vi "Handle Filling.vi"(8 "error in (no error)":errorcluster, 11 "Stand in":refnum<class "Stand.lvclass">) -> (0 "error out":errorcluster, 3 "Stand out":refnum<class "Stand.lvclass">)   [LabVIEW 2019, in "Stand.lvclass"]
uses:
  Stand.lvclass
  D:/GIT H4000/H4000/src/Device_class/Device.lvclass
  Stand.lvclass/Stand.ctl
  Device_class/Device.lvclass/Device.ctl
  FPGA/TypeDef/DO index.ctl
  TypeDef/Direction.ctl
  FPGA/TypeDef/AI index.ctl
  AI_class/AI.lvclass/AI.ctl
  AnalogComparator_class/AnalogComparator.lvclass/AnalogComparator.ctl
  TypeDef/Step_Name.ctl
  TypeDef/Active Motor.ctl
  TypeDef/Motor N.ctl
  f638fa31-f737-482a-bde8-81f5a2056bae.vi
  AnalogComparator_class/GetStatus.vi
  FPGA_API_class/FPGA API.lvclass
  Device_class/Device.lvclass
  PM_Group_class/PM_Group.lvclass
  AI_class/AI.lvclass
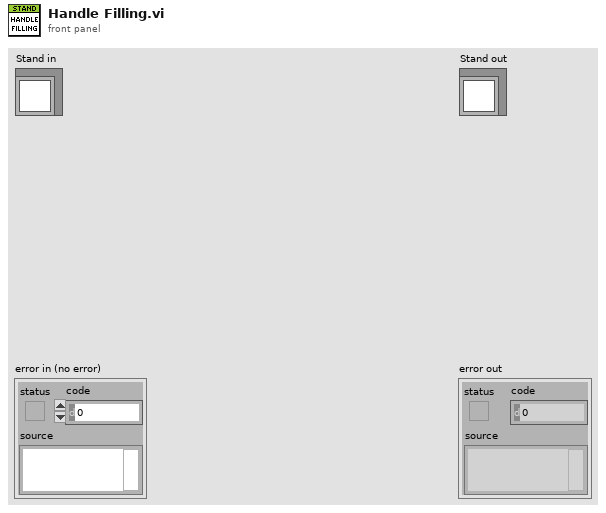
[diagram p1: front panel]
types:
  T1 = typedef "Step_Name.ctl" = enum16{"NONE", "Filling DUT", "Filling Chamber", "Pressure Up DUT", "Abrupt Pressure Release DUT", "Smooth Pressure Release DUT", "Pressure Up Chamber", "Abrupt Pressure Release Chamber", "Smooth Pressure Release Chamber", "Measuring leakage sensor 41.3", "Measuring leakage burette 42", "Low Pressure DUT", "Low Pressure Chamber", "Low Pressure HPP", "ALARM", "Open Air", "MicroStep DUT", "MicroStep CMBR"}
  T2 = typedef "Direction.ctl" = enum16{"None", "Chamber", "DUT"}
  T3 = typedef "Active Motor.ctl" = cluster{"Active":bool, "MotorN":T4}
  T4 = typedef "Motor N.ctl" = enum16{"M12", "M21", "M24"}
  T5 = typedef "AI index.ctl" = u8
  T6 = typedef "DO index.ctl" = u8
  T7 = typedef "AI_Data.ctl" = cluster{"Stat Data":T8, "OutOfRangeMax":bool, "OutOfRangeMin":bool, "HIHI":bool, "HI":bool, "LO":bool, "LOLO":bool}
  T8 = typedef "AI Statistics Data.ctl" = cluster{"raw mean":dbl, "scl mean":dbl, "raw mean 1Hz":dbl, "scl mean 1Hz":dbl, "raw standard deviation":dbl, "raw max value":dbl, "raw min value":dbl}
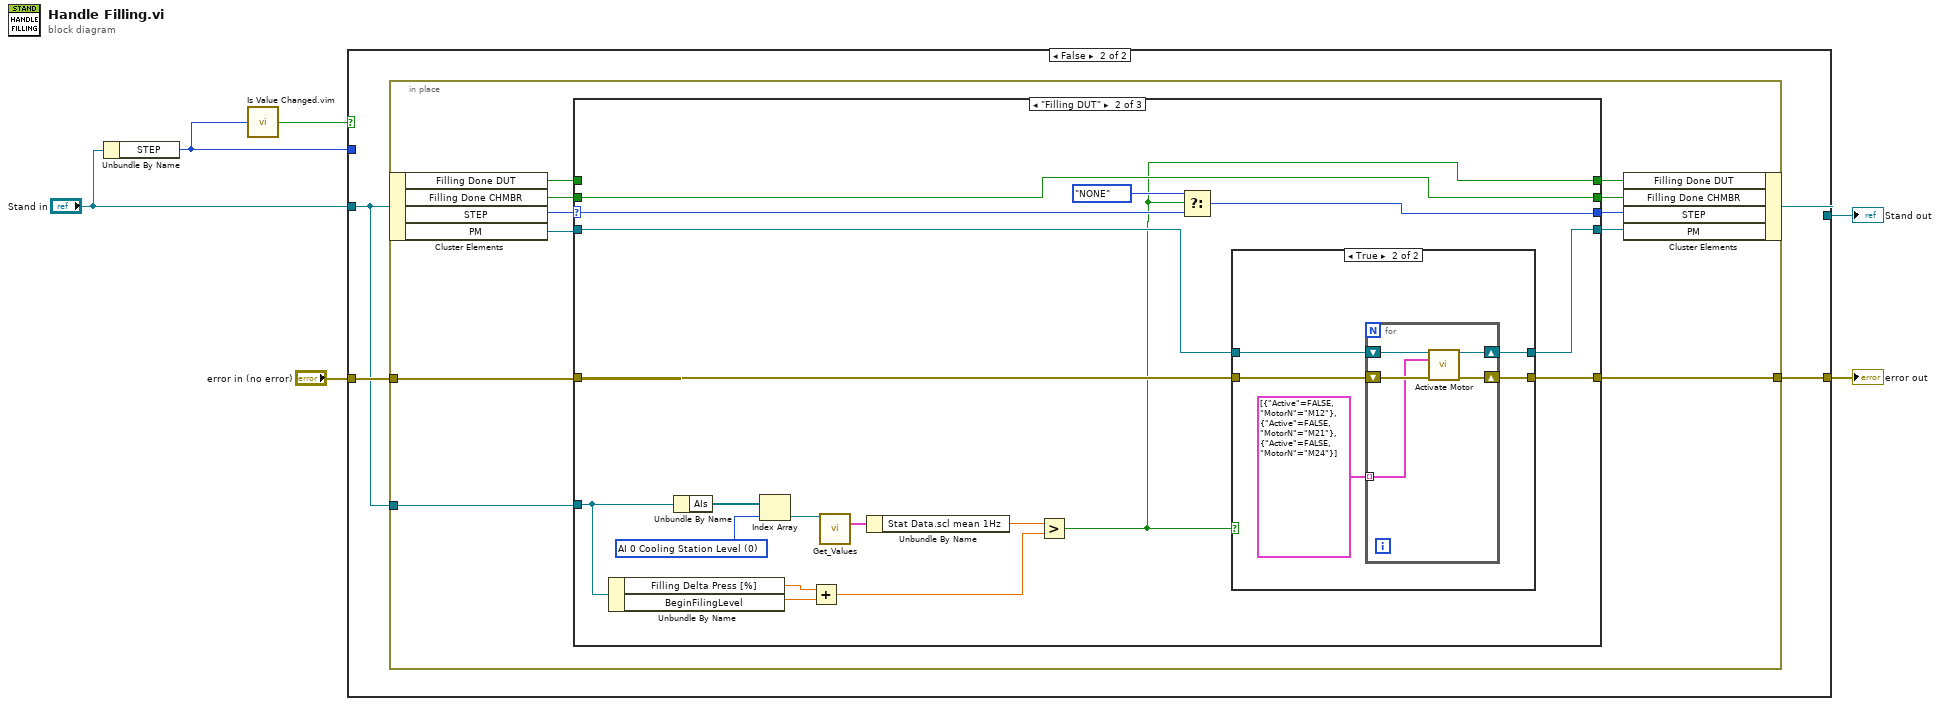
[diagram p0: block diagram]
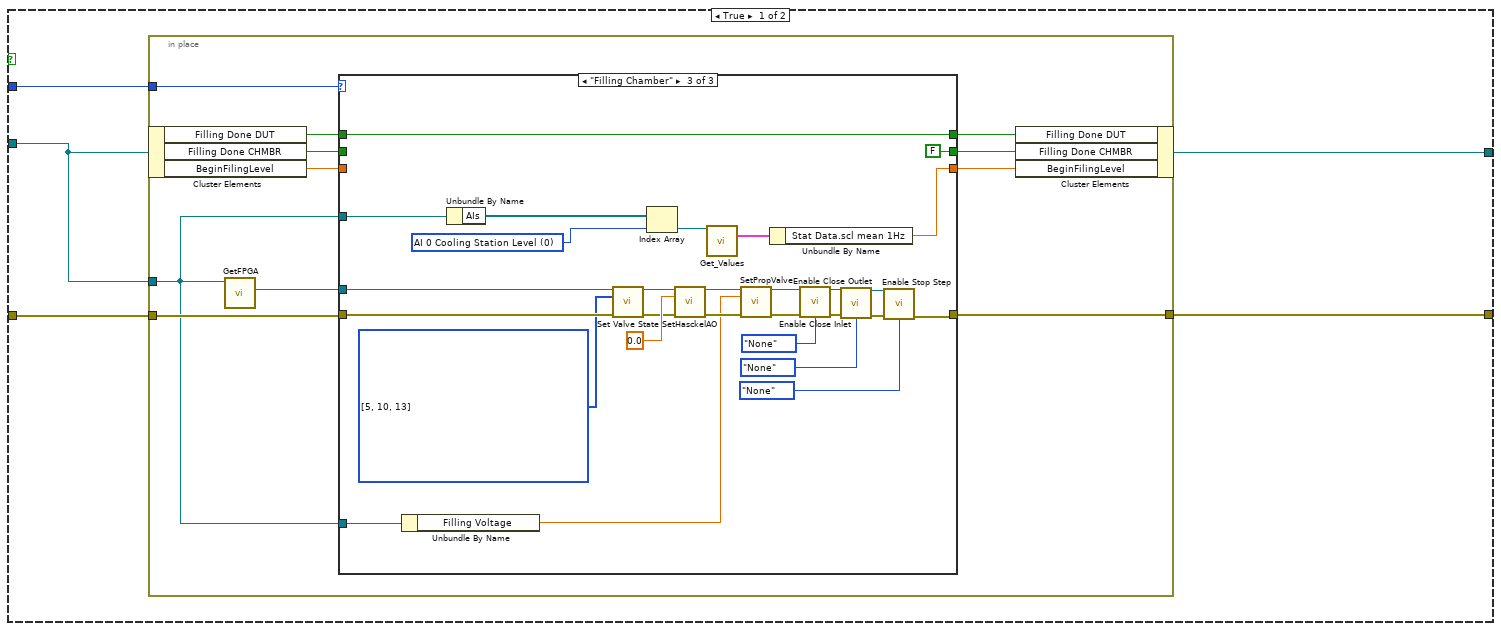
[diagram p2: hidden frame]
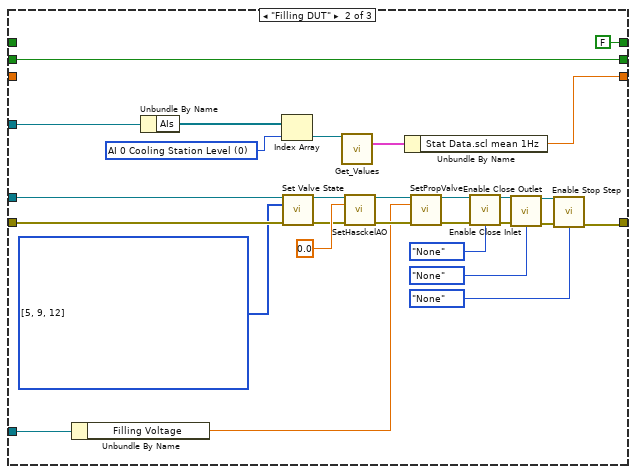
[diagram p4: hidden frame]
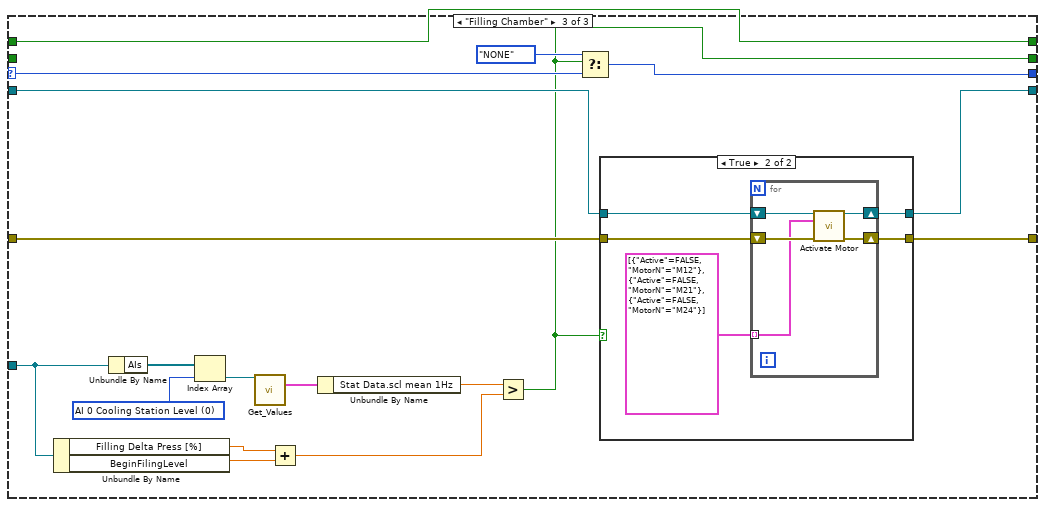
[diagram p7: hidden frame]
diagram:
  n1 = Unbundle By Name("Stand in") -> ("STEP"=w1:T1)
  n2 = call "Is Value Changed.vim"("value"=w1) -> ("changed or first call?"=w6:bool)
  n3 = case shown="False" w6 {
    tunnel: w1 -> [w11 _]
    tunnel: "Stand in" -> [w9 w85]
    tunnel: "error in (no error)" -> [w10 w86]
    tunnel: [w8 w84] -> w5
    tunnel: [w7 w83] -> w4
    frame True {
      n4 = in-place {
        in-place-border: w11 -> [w22]
        in-place-border: [w21] -> w7
        in-place-border: w10 -> [w20]
        in-place-border: w9 -> [w18]
        n5 = in-place-cluster #1(w9) -> ("Filling Done DUT"=w14:bool, "Filling Done CHMBR"=w13:bool, "BeginFilingLevel"=w17:dbl)
        n6 = call "GetFPGA.vi"("Device in"=w18) -> ("FPGA API.lvclass"=w19:refnum<class "FPGA API.lvclass">)  [unwired: 10 in]
        n7 = case shown="\"Filling Chamber\"" w22 {
          tunnel: w20 -> [w26 w54 w82]
          tunnel: [w26 w36 w65] -> w21
          tunnel: w19 -> [_ w47 w76]
          tunnel: w18 -> [_ w46 w75]
          tunnel: w18 -> [_ w30 w58]
          tunnel: w17 -> [w25 _ _]
          tunnel: [w25 w29 w57] -> w16
          tunnel: [w24 FALSE ("Filling Done DUT") w56] -> w15
          tunnel: w14 -> [w24 _ w56]
          tunnel: w13 -> [w23 w27 _]
          tunnel: [w23 w27 FALSE ("Filling Done CHMBR")] -> w12
          frame Default {
          }
          frame "Filling DUT" {
            w31 = T5 0 items=["AI 0 Cooling Station Level", "AI 1 Cooling Station Temp", "AI 2 Oil Supply Level", "AI 3 Oil Supply Temp", "AI 4 ", "AI 5 Pressure Haskel", "AI 6 Pressure DUT", "AI 7 Pressure Chamber", "AI 8 Pressure Air inlet", "AI 9 Pressure Air outlet", "AI 10 Pressure Messure Line"] ("AI index")
            w48 = T6[] [5, 9, 12] items=["DO 0 [KP1] [M12]", "DO 1 [ON KP2] [M21]", "DO 2 [ON KP3] [M24]", "DO 3 [WATER Y18.1 [DO3]]", "DO 4 [WATER Y18.2 [DO4]]", "DO 5 [KP6 Y29.1 33.7]", "DO 6 [KP7 Y29.2 33.8]", "DO 7 [KP8 Y29.3 33.9]", "DO 8 [KP9 Y29.4  33.12]", "DO 9 [KP10 Y29.5 33.1]", "DO 10 [KP11 Y29.6 33.2]", "DO 11 [KP12 Y29.7  33.13]", "DO 12 [KP13 Y29.8  33.11]", "DO 13 [KP14 Y29.9 33.10]", "DO 14 [KP15 Y29.10  33.6]", "DO 15 [KP16 Y29.11  33.5]", "DO 16 [KP17 Y29.12  33.4]", "DO 17 [KP18 Y29.13 33.3]", "DO 18 [AIR KP19]", "DO 19 [STEP DRIVE EN KP20]", "DO 20 [KP21 Y44.1 OPEN]", "DO 21 [ KP22 Y44.1 CLOSE]", "DO 22 [ KP23 Y44.2 OPEN]", "DO 23", "DO 24 [STEP DRIVE 1]", "DO 25 [STEP DRIVE 2]"] ("#DO")
            n8 = Unbundle By Name(w46) -> ("Filling Voltage"=w45:dbl)
            n9 = Unbundle By Name(w30) -> ("AIs"=w34:refnum<class "AI.lvclass">[])
            n10 = Index Array(array=w34, index=w31) -> (element=w33:refnum<class "AI.lvclass">)
            n11 = call "Set Valve State.vi"("reference in"=w47, "#DO"=w48, "error in (no error)"=w54) -> ("reference out"=w53:refnum<class "FPGA API.lvclass">, "error out"=w51:errorcluster)  [unwired: 11 in]
            n12 = call "Get_Values.vi"("reference in"=w33) -> ("Data"=w32:T7)  [unwired: 14 in]
            n13 = call-dynamic "SetHasckelAO.vi"("FPGA API in"=w53, "Haskel in"=0.0, "error in (no error)"=w51) -> ("FPGA API out"=w50:refnum<class "FPGA API.lvclass">, "error out"=w49:errorcluster)  [unwired: 11 in]
            n14 = Unbundle By Name(w32) -> ("Stat Data.scl mean 1Hz"=w29:dbl)
            n15 = call-dynamic "SetPropValve.vi"("FPGA API in"=w50, "AO 1"=w45, "error in (no error)"=w49) -> ("FPGA API out"=w44:refnum<class "FPGA API.lvclass">, "error out"=w43:errorcluster)  [unwired: 11 in]
            n16 = call-dynamic "Enable Close Inlet.vi"("FPGA API in"=w44, "error in (no error)"=w43, "Direction"=Direction."None") -> ("FPGA API out"=w41:refnum<class "FPGA API.lvclass">, "error out"=w40:errorcluster)  [unwired: 11 in]
            n17 = call-dynamic "Enable Close Outlet.vi"("FPGA API in"=w41, "error in (no error)"=w40, "Direction"=Direction."None") -> ("FPGA API out"=w38:refnum<class "FPGA API.lvclass">, "error out"=w37:errorcluster)  [unwired: 11 in]
            n18 = call-dynamic "Enable Stop Step.vi"("FPGA API in"=w38, "error in (no error)"=w37, "Direction"=Direction."None") -> ("error out"=w36:errorcluster)  [unwired: 11 in, 1 out]
          }
          frame "Filling Chamber" {
            w59 = T5 0 items=["AI 0 Cooling Station Level", "AI 1 Cooling Station Temp", "AI 2 Oil Supply Level", "AI 3 Oil Supply Temp", "AI 4 ", "AI 5 Pressure Haskel", "AI 6 Pressure DUT", "AI 7 Pressure Chamber", "AI 8 Pressure Air inlet", "AI 9 Pressure Air outlet", "AI 10 Pressure Messure Line"] ("AI index")
            w63 = T6[] [5, 10, 13] items=["DO 0 [KP1] [M12]", "DO 1 [ON KP2] [M21]", "DO 2 [ON KP3] [M24]", "DO 3 [WATER Y18.1 [DO3]]", "DO 4 [WATER Y18.2 [DO4]]", "DO 5 [KP6 Y29.1 33.7]", "DO 6 [KP7 Y29.2 33.8]", "DO 7 [KP8 Y29.3 33.9]", "DO 8 [KP9 Y29.4  33.12]", "DO 9 [KP10 Y29.5 33.1]", "DO 10 [KP11 Y29.6 33.2]", "DO 11 [KP12 Y29.7  33.13]", "DO 12 [KP13 Y29.8  33.11]", "DO 13 [KP14 Y29.9 33.10]", "DO 14 [KP15 Y29.10  33.6]", "DO 15 [KP16 Y29.11  33.5]", "DO 16 [KP17 Y29.12  33.4]", "DO 17 [KP18 Y29.13 33.3]", "DO 18 [AIR KP19]", "DO 19 [STEP DRIVE EN KP20]", "DO 20 [KP21 Y44.1 OPEN]", "DO 21 [ KP22 Y44.1 CLOSE]", "DO 22 [ KP23 Y44.2 OPEN]", "DO 23", "DO 24 [STEP DRIVE 1]", "DO 25 [STEP DRIVE 2]"] ("#DO")
            n19 = Unbundle By Name(w75) -> ("Filling Voltage"=w74:dbl)
            n20 = Unbundle By Name(w58) -> ("AIs"=w62:refnum<class "AI.lvclass">[])
            n21 = call "Set Valve State.vi"("reference in"=w76, "#DO"=w63, "error in (no error)"=w82) -> ("reference out"=w81:refnum<class "FPGA API.lvclass">, "error out"=w79:errorcluster)  [unwired: 11 in]
            n22 = Index Array(array=w62, index=w59) -> (element=w61:refnum<class "AI.lvclass">)
            n23 = call-dynamic "SetHasckelAO.vi"("FPGA API in"=w81, "Haskel in"=0.0, "error in (no error)"=w79) -> ("FPGA API out"=w78:refnum<class "FPGA API.lvclass">, "error out"=w77:errorcluster)  [unwired: 11 in]
            n24 = call "Get_Values.vi"("reference in"=w61) -> ("Data"=w60:T7)  [unwired: 14 in]
            n25 = call-dynamic "SetPropValve.vi"("FPGA API in"=w78, "AO 1"=w74, "error in (no error)"=w77) -> ("FPGA API out"=w73:refnum<class "FPGA API.lvclass">, "error out"=w72:errorcluster)  [unwired: 11 in]
            n26 = Unbundle By Name(w60) -> ("Stat Data.scl mean 1Hz"=w57:dbl)
            n27 = call-dynamic "Enable Close Inlet.vi"("FPGA API in"=w73, "error in (no error)"=w72, "Direction"=Direction."None") -> ("FPGA API out"=w70:refnum<class "FPGA API.lvclass">, "error out"=w69:errorcluster)  [unwired: 11 in]
            n28 = call-dynamic "Enable Close Outlet.vi"("FPGA API in"=w70, "error in (no error)"=w69, "Direction"=Direction."None") -> ("FPGA API out"=w67:refnum<class "FPGA API.lvclass">, "error out"=w66:errorcluster)  [unwired: 11 in]
            n29 = call-dynamic "Enable Stop Step.vi"("FPGA API in"=w67, "error in (no error)"=w66, "Direction"=Direction."None") -> ("error out"=w65:errorcluster)  [unwired: 11 in, 1 out]
          }
        }
        n30 = in-place-cluster #1("Filling Done DUT"=w15, "Filling Done CHMBR"=w12, "BeginFilingLevel"=w16) -> (w8:refnum<class "Stand.lvclass">)
      }
    }
    frame False {
      n31 = in-place {
        in-place-border: [w97] -> w83
        in-place-border: w86 -> [w96]
        in-place-border: w85 -> [w93]
        n32 = in-place-cluster #2(w85) -> ("Filling Done DUT"=w89:bool, "Filling Done CHMBR"=w90:bool, "STEP"=w91:T1, "PM"=w95:refnum<class "PM_Group.lvclass">)
        n33 = case shown="\"Filling DUT\"" w91 {
          selector: w91 -> [w100 w111 w141]
          tunnel: w96 -> [w102 w107 w137]
          tunnel: [w102 w106 w136] -> w97
          tunnel: w95 -> [w101 w109 w139]
          tunnel: [w101 w108 w138] -> w94
          tunnel: w93 -> [_ w105 w135]
          tunnel: [w100 w110 w140] -> w92
          tunnel: w90 -> [w99 w104 _]
          tunnel: w89 -> [w98 _ w134]
          tunnel: [w99 w104 w133] -> w88
          tunnel: [w98 w103 w134] -> w87
          frame Default {
          }
          frame "Filling DUT" {
            w118 = T5 0 items=["AI 0 Cooling Station Level", "AI 1 Cooling Station Temp", "AI 2 Oil Supply Level", "AI 3 Oil Supply Temp", "AI 4 ", "AI 5 Pressure Haskel", "AI 6 Pressure DUT", "AI 7 Pressure Chamber", "AI 8 Pressure Air inlet", "AI 9 Pressure Air outlet", "AI 10 Pressure Messure Line"] ("AI index")
            n34 = Unbundle By Name(w105) -> ("Filling Delta Press [%]"=w116:dbl, "BeginFilingLevel"=w115:dbl)
            n35 = Unbundle By Name(w105) -> ("AIs"=w117:refnum<class "AI.lvclass">[])
            n36 = Index Array(array=w117, index=w118) -> (element=w119:refnum<class "AI.lvclass">)
            n37 = Add(x=w116, y=w115) -> (x+y=w113:dbl)
            n38 = call "Get_Values.vi"("reference in"=w119) -> ("Data"=w120:T7)  [unwired: 14 in]
            n39 = Unbundle By Name(w120) -> ("Stat Data.scl mean 1Hz"=w114:dbl)
            n40 = Greater?(x=w114, y=w113) -> (0:w103:bool)
            n41 = Select(t=Step_Name."NONE" ("stepName"), s=w103, f=w111) -> (s? t:f=w110:T1)
            n42 = case shown="True" w103 {
              tunnel: w109 -> [w121 w126]
              tunnel: [w121 w125] -> w108
              tunnel: w107 -> [w122 w124]
              tunnel: [w122 w123] -> w106
              frame False {
              }
              frame True {
                n43 = for {
                  tunnel: T3[] [{"Active"=FALSE, "MotorN"=enum."M12"}, {"Active"=FALSE, "MotorN"=enum."M21"}, {"Active"=FALSE, "MotorN"=enum."M24"}] ("Array") -> [w130] mode=indexing
                  shift-right: [w129] -> w125
                  shift-left: w126 -> [w132]
                  shift-right: [w128] -> w123
                  shift-left: w124 -> [w131]
                  n44 = call "Activate Motor.vi"("reference in"=w132, "Active Motor"=w130, "error in (no error)"=w131) -> ("reference out"=w129:refnum<class "PM_Group.lvclass">, "error out"=w128:errorcluster)  [unwired: 11 in]
                }
              }
            }
          }
          frame "Filling Chamber" {
            w148 = T5 0 items=["AI 0 Cooling Station Level", "AI 1 Cooling Station Temp", "AI 2 Oil Supply Level", "AI 3 Oil Supply Temp", "AI 4 ", "AI 5 Pressure Haskel", "AI 6 Pressure DUT", "AI 7 Pressure Chamber", "AI 8 Pressure Air inlet", "AI 9 Pressure Air outlet", "AI 10 Pressure Messure Line"] ("AI index")
            n45 = Unbundle By Name(w135) -> ("Filling Delta Press [%]"=w146:dbl, "BeginFilingLevel"=w145:dbl)
            n46 = Unbundle By Name(w135) -> ("AIs"=w147:refnum<class "AI.lvclass">[])
            n47 = Index Array(array=w147, index=w148) -> (element=w149:refnum<class "AI.lvclass">)
            n48 = call "Get_Values.vi"("reference in"=w149) -> ("Data"=w150:T7)  [unwired: 14 in]
            n49 = Add(x=w146, y=w145) -> (x+y=w143:dbl)
            n50 = Unbundle By Name(w150) -> ("Stat Data.scl mean 1Hz"=w144:dbl)
            n51 = Greater?(x=w144, y=w143) -> (0:w133:bool)
            n52 = Select(t=Step_Name."NONE" ("stepName"), s=w133, f=w141) -> (s? t:f=w140:T1)
            n53 = case shown="True" w133 {
              tunnel: w139 -> [w151 w156]
              tunnel: [w151 w155] -> w138
              tunnel: w137 -> [w152 w154]
              tunnel: [w152 w153] -> w136
              frame False {
              }
              frame True {
                n54 = for {
                  tunnel: T3[] [{"Active"=FALSE, "MotorN"=enum."M12"}, {"Active"=FALSE, "MotorN"=enum."M21"}, {"Active"=FALSE, "MotorN"=enum."M24"}] ("Array") -> [w160] mode=indexing
                  shift-right: [w159] -> w155
                  shift-left: w156 -> [w162]
                  shift-right: [w158] -> w153
                  shift-left: w154 -> [w161]
                  n55 = call "Activate Motor.vi"("reference in"=w162, "Active Motor"=w160, "error in (no error)"=w161) -> ("reference out"=w159:refnum<class "PM_Group.lvclass">, "error out"=w158:errorcluster)  [unwired: 11 in]
                }
              }
            }
          }
        }
        n56 = in-place-cluster #2("Filling Done DUT"=w87, "Filling Done CHMBR"=w88, "STEP"=w92, "PM"=w94) -> (w84:refnum<class "Stand.lvclass">)
      }
    }
  }
  "error out" <- w4
  "Stand out" <- w5
